vi "stop.vi"(8 "error in (no error)":errorcluster, 10 "Stop":bool, 11 "AndorIKonAcquisitor in":refnum<class "AndorIKonAcquisitor.lvclass">) -> (0 "error out":errorcluster, 2 "Stopped":bool=TRUE, 3 "AndorIKonAcquisitor out":refnum<class "AndorIKonAcquisitor.lvclass">)   [LabVIEW 2011, in "Hardware.lvlib" / "Channels.lvlib" / "AndorIKonAcquisitor.lvclass"]
uses:
  AndorIKonAcquisitor.lvclass
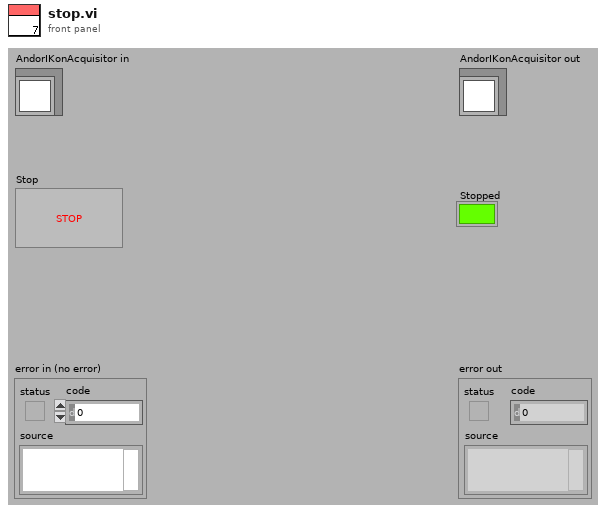
[diagram p1: front panel]
types:
  T1 = typedef "Error Code Enum typedef.ctl" = enum32{"N/A (0)", "DRV_ERROR_CODES", "DRV_SUCCESS", "DRV_VXDNOTINSTALLED", "DRV_ERROR_SCAN", "DRV_ERROR_CHECK_SUM", "DRV_ERROR_FILELOAD", "DRV_UNKNOWN_FUNC", "DRV_ERROR_VXD_INIT", "DRV_ERROR_ADDRESS", "DRV_ERROR_PAGELOCK", "DRV_ERROR_PAGEUNLOCK", "DRV_ERROR_BOARDTEST", "DRV_ERROR_ACK", "DRV_ERROR_UP_FIFO", "DRV_ERROR_PATTERN", "N/A (16)", "DRV_ACQUISITION_ERRORS", "DRV_ACQ_BUFFER", "DRV_ACQ_DOWNFIFO_FULL", "DRV_PROC_UNKONWN_INSTRUCTION", "DRV_ILLEGAL_OP_CODE", "DRV_KINETIC_TIME_NOT_MET", "DRV_ACCUM_TIME_NOT_MET", "DRV_NO_NEW_DATA", "N/A (25)", "DRV_SPOOLERROR", "N/A (27)", "N/A (28)", "N/A (29)", "N/A (30)", "N/A (31)", "N/A (32)", "DRV_TEMPERATURE_CODES", "DRV_TEMPERATURE_OFF", "DRV_TEMPERATURE_NOT_STABILIZED", "DRV_TEMPERATURE_STABILIZED", "DRV_TEMPERATURE_NOT_REACHED", "DRV_TEMPERATURE_OUT_RANGE", "DRV_TEMPERATURE_NOT_SUPPORTED", "DRV_TEMPERATURE_DRIFT", "N/A (41)", "N/A (42)", "N/A (43)", "N/A (44)", "N/A (45)", "N/A (46)", "N/A (47)", "N/A (48)", "DRV_GENERAL_ERRORS", "DRV_INVALID_AUX", "DRV_COF_NOTLOADED", "DRV_FPGAPROG", "DRV_FLEXERROR", "DRV_GPIBERROR", "N/A (55)", "N/A (56)", "N/A (57)", "N/A (58)", "N/A (59)", "N/A (60)", "N/A (61)", "N/A (62)", "N/A (63)", "DRV_DATATYPE", "DRV_DRIVER_ERRORS", "DRV_P1INVALID", "DRV_P2INVALID", "DRV_P3INVALID", "DRV_P4INVALID", "DRV_INIERROR", "DRV_COFERROR", "DRV_ACQUIRING", "DRV_IDLE", "DRV_TEMPCYCLE", "DRV_NOT_INITIALIZED", "DRV_P5INVALID", "DRV_P6INVALID", "DRV_INVALID_MODE", "DRV_INVALID_FILTER", "DRV_I2CERRORS", "DRV_I2CDEVNOTFOUND", "DRV_I2CTIMEOUT", "DRV_P7INVALID", "N/A (84)", "N/A (85)", "N/A (86)", "N/A (87)", "N/A (88)", "N/A (89)", "DRV_IOCERROR", "DRV_VRMVERSIONERROR"}
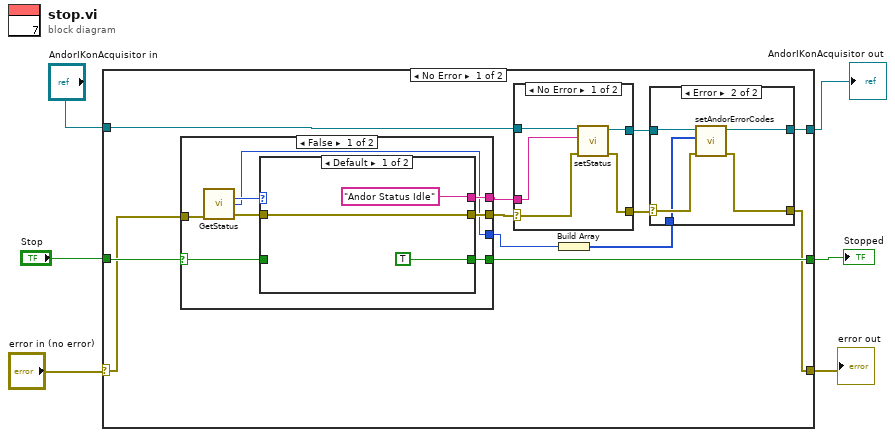
[diagram p0: block diagram]
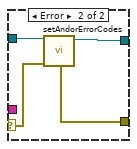
[diagram p3: hidden frame]
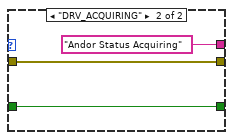
[diagram p4: hidden frame]
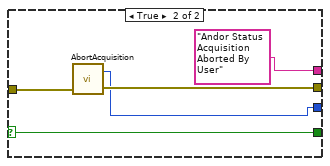
[diagram p5: hidden frame]
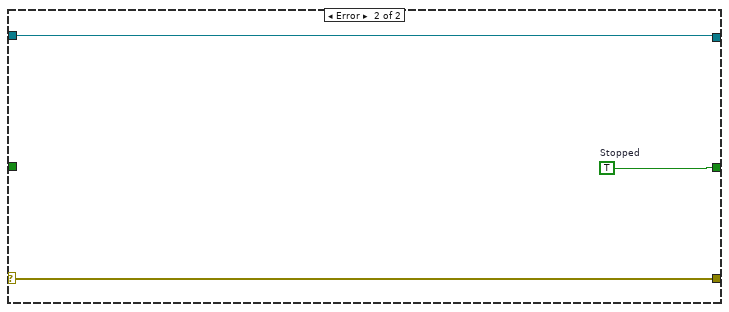
[diagram p6: hidden frame]
diagram:
  n1 = case shown="No Error" "error in (no error)" {
    selector: "error in (no error)" -> [w17 w56]
    tunnel: "AndorIKonAcquisitor in" -> [w13 w55]
    tunnel: [w7 w56] -> w4
    tunnel: [w8 w55] -> w3
    tunnel: "Stop" -> [w18 _]
    tunnel: [w16 w54] -> w1
    frame No Error {
      n2 = case shown="False" w18 {
        selector: w18 -> [w39 w53]
        tunnel: w17 -> [w42 w51]
        tunnel: [w37 w50] -> w15
        tunnel: [w38 w53] -> w16
        tunnel: [w36 "Andor Status Acquisition Aborted By User"] -> w14
        tunnel: [w35 w49] -> w10
        frame False {
          n3 = call <userlib>:"GetStatus.vi"("error in (no error)"=w42) -> ("error out"=w40:errorcluster, "DLL error code"=w35:u32, "status"=w41:T1)  [unwired: 2 in]
          n4 = case shown="Default" w41 {
            tunnel: w40 -> [w44 w47]
            tunnel: [TRUE w48] -> w38
            tunnel: w39 -> [_ w48]
            tunnel: [w44 w47] -> w37
            tunnel: ["Andor Status Idle" "Andor Status Acquiring"] -> w36
            frame Default {
            }
            frame "DRV_ACQUIRING" {
            }
          }
        }
        frame True {
          n5 = call <userlib>:"AbortAcquisition.vi"("error in (no error)"=w51) -> ("error out"=w50:errorcluster, "DLL error code"=w49:u32)  [unwired: 1 in]
        }
      }
      n6 = case shown="No Error" w15 {
        selector: w15 -> [w27 w33]
        tunnel: w13 -> [w30 w34]
        tunnel: [w29 w31] -> w12
        tunnel: [w28 w32] -> w11
        tunnel: w14 -> [w26 _]
        frame No Error {
          n7 = call-dynamic "setStatus.vi"("error in (no error)"=w27, "Status"=w26, "CameraAcquisitor.lvclass in"=w30) -> ("error out"=w28:errorcluster, "CameraAcquisitor.lvclass out"=w29:refnum<class "AndorIKonAcquisitor.lvclass">)  [unwired: 7 in]
        }
        frame Error {
          n8 = call-dynamic "setAndorErrorCodes.vi"("error in (no error)"=w33, "AndorIKonAcquisitor.lvclass in"=w34) -> ("error out"=w32:errorcluster, "AndorIKonAcquisitor.lvclass out"=w31:refnum<class "AndorIKonAcquisitor.lvclass">)  [unwired: 8 in]
        }
      }
      n9 = Build Array(w10) -> (w9:u32[])
      n10 = case shown="Error" w11 {
        selector: w11 -> [w20 w25]
        tunnel: [w20 w24] -> w7
        tunnel: w12 -> [w19 w23]
        tunnel: w9 -> [_ w22]
        tunnel: [w19 w21] -> w8
        frame No Error {
        }
        frame Error {
          n11 = call-dynamic "setAndorErrorCodes.vi"("error in (no error)"=w25, "Andor Error Codes"=w22, "AndorIKonAcquisitor.lvclass in"=w23) -> ("error out"=w24:errorcluster, "AndorIKonAcquisitor.lvclass out"=w21:refnum<class "AndorIKonAcquisitor.lvclass">)  [unwired: 7 in]
        }
      }
    }
    frame Error {
      w54 = TRUE  # Stopped
    }
  }
  "error out" <- w4
  "AndorIKonAcquisitor out" <- w3
  "Stopped" <- w1
